vi "Day 6 (Part Two).vi"() -> ()   [LabVIEW 2021]
panel:
  out "Position":i32
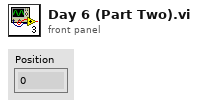
[diagram p1: front panel]
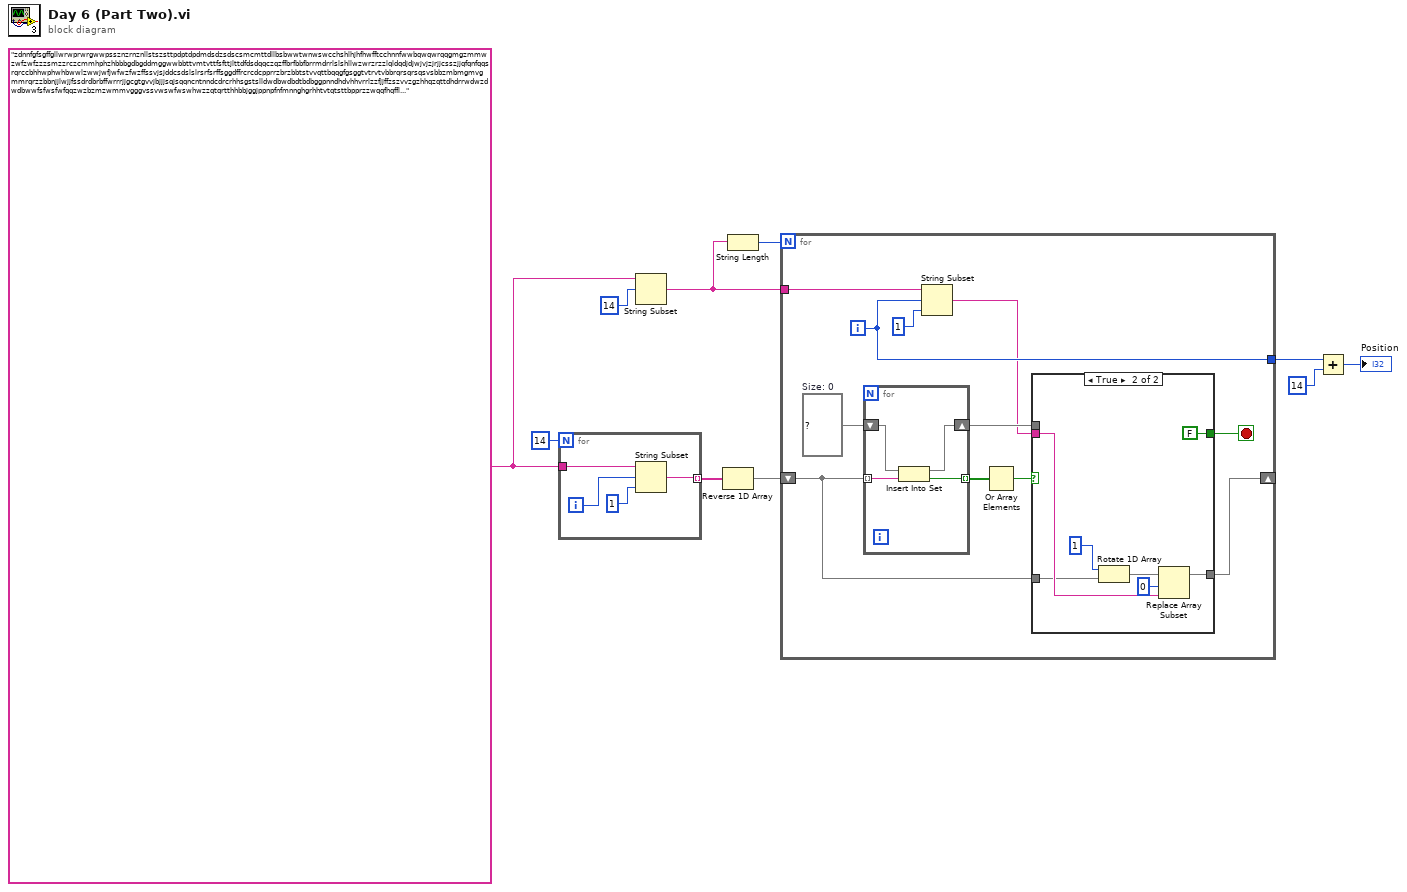
[diagram p0: block diagram]
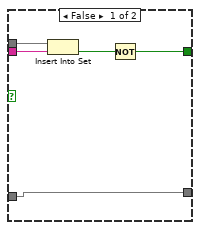
[diagram p2: hidden frame]
diagram:
  w1 = "zdnnfgfsgffgllwrwprwrgwwpssznzrnznllstszsttpdptdpdmdsdzsdscsmcmttdllbsbwwtwnwswcchshlhjhfhwfftcchnnfwwbqwqwrqqgmgzmmwzwfzwfzzzsmzzrczcmmhphzhbbbgdbgddmggwwbbttvmtvttfsfttjlttdfdsdqqczqzffbrfbbfbrrmdrrlslshllwzwrzrzzlqldqdjdjwjvjzjrjjcsszjjqfqnfqqsrqrccbhhwphwhbwwlzwwjwfjwfwzfwzffssvjsjddcsdslslrsrfsrffsggdffrcrcdcpprrzbrzbbtstvvqttbqqgfgsggtvtrvtvbbrqrsqrsqsvsbbzmbmgmvgmmrqrzzbbnjjlwjjfssdrdbrbffwrrrjjgcgtgvvjbjjjsqjsqqncntnndcdrcrhhsgstslldwdbwdbdtbdbggpnndhdvhhvrrlzzfjjffzszvvzgzhhqzqttdhdrrwdwzdwdbwwfsfwsfwfqqzwzbzmzwmmvgggvssvwswfwswhwzzqtqrtthhbbjggjppnpfnfmnnghgrhhtvtqtsttbpprzzwqqfhqffl..."
  n1 = for {
    N: 14 -> [_]
    tunnel: w1 -> [w14]
    tunnel: [w11] -> w4 mode=indexing
    i -> [w13]
    n2 = String Subset(string=w14, offset (0)=w13, length (rest)=1 ("length (rest)")) -> (substring=w11:string)
  }
  n3 = String Subset(string=w1, offset (0)=14) -> (substring=w8:string)  [unwired: 1 in]
  n4 = Reverse 1D Array(array=w4) -> (reversed array=w2:string[])
  n5 = String Length(string=w8) -> (length=w7:i32)
  n6 = for {
    N: w7 -> [_]
    tunnel: w8 -> [w25]
    tunnel: [w23] -> w6
    shift-right: [w15] -> _
    shift-left: w2 -> [w16]
    i -> [w23]
    stop <- w17 stop-if-true
    w22 = set{string} {}  # Size: 0
    n7 = for {
      tunnel: w16 -> [w41] mode=indexing
      shift-right: [w39] -> w19
      shift-left: w22 -> [w40]
      tunnel: [w38] -> w21 mode=indexing
      n8 = Insert Into Set(10:w41, 11:w40) -> (2:w38:bool, 3:w39:set{string})
    }
    n9 = String Subset(string=w25, offset (0)=w23, length (rest)=1 ("length (rest)")) -> (substring=w18:string)
    n10 = Or Array Elements(Boolean array=w21) -> (logical OR=w20:bool)
    n11 = case shown="True" w20 {
      tunnel: w19 -> [w30 _]
      tunnel: w18 -> [w29 w37]
      tunnel: [w27 FALSE] -> w17
      tunnel: w16 -> [w26 w34]
      tunnel: [w26 w32] -> w15
      frame False {
        n12 = Insert Into Set(10:w29, 11:w30) -> (2:w28:bool)  [unwired: 1 out]
        n13 = Not(x=w28) -> (.not. x?=w27:bool)
      }
      frame True {
        n14 = Rotate 1D Array(1:w34, 2:1 ("n")) -> (0:w33:string[])
        n15 = Replace Array Subset(array=w33, new element=w37, index=0) -> (w32:string[])
      }
    }
  }
  n16 = Add(x=w6, y=14) -> (x+y=→"Position":i32)
